vi "Divby3.vi"() -> ()   [LabVIEW 2020]
panel:
  out "Odd numbers divisible by 3":dbl[](array[numeric])
  out "Even numbers divisible by 3":dbl[](array[numeric])
  in  "Temp":dbl[](array[numeric])
  in  "Input  Array":dbl[](array[numeric])
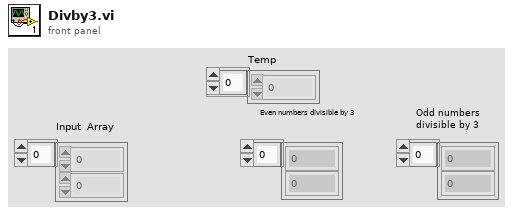
[diagram p1: front panel]
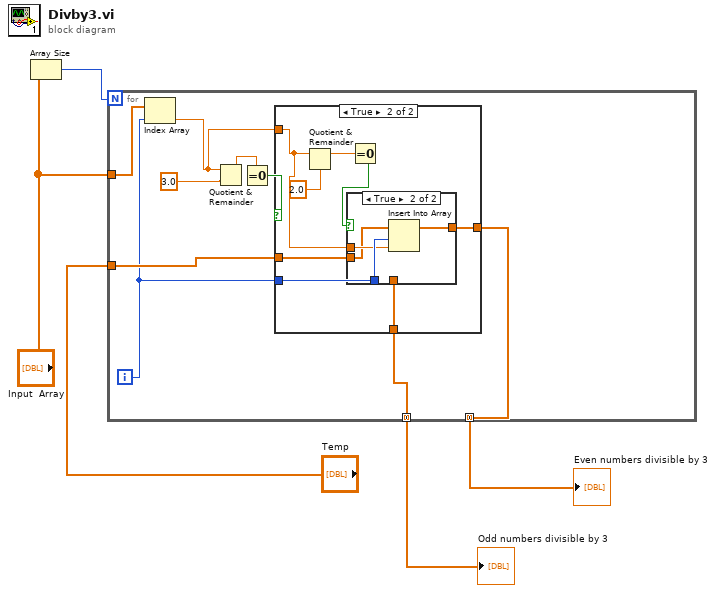
[diagram p0: block diagram]
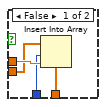
[diagram p3: hidden frame]
diagram:
  n1 = Array Size(array="Input  Array") -> (size(s)=w5:i32)
  n2 = for {
    N: w5 -> [_]
    tunnel: "Input  Array" -> [w14]
    tunnel: "Temp" -> [w9]
    tunnel: [w7] -> w2 mode=concatenating
    tunnel: [w6] -> w1 mode=concatenating
    i -> [w8]
    n3 = Index Array(array=w14, index=w8) -> (element=w10:dbl)
    n4 = Quotient & Remainder(x=w10, y=3.0) -> (x-y*floor(x/y)=w12:dbl)  [unwired: 1 out]
    n5 = Equal To 0?(x=w12) -> (x = 0?=w11:bool)
    n6 = case shown="True" w11 {
      tunnel: w10 -> [_ w17]
      tunnel: w9 -> [_ w19]
      tunnel: w8 -> [_ w18]
      tunnel: [_ w16] -> w7
      tunnel: [_ w15] -> w6
      frame False {
      }
      frame True {
        n7 = Quotient & Remainder(x=w17, y=2.0) -> (x-y*floor(x/y)=w21:dbl)  [unwired: 1 out]
        n8 = Equal To 0?(x=w21) -> (x = 0?=w20:bool)
        n9 = case shown="True" w20 {
          tunnel: w19 -> [w23 w27]
          tunnel: w18 -> [w24 w30]
          tunnel: w17 -> [w26 w29]
          tunnel: [w25 _] -> w16
          tunnel: [_ w28] -> w15
          frame False {
            n10 = Insert Into Array(array=w23, index=w24, new element=w26) -> (w25:dbl[])
          }
          frame True {
            n11 = Insert Into Array(array=w27, index=w30, new element=w29) -> (w28:dbl[])
          }
        }
      }
    }
  }
  "Even numbers divisible by 3" <- w1
  "Odd numbers divisible by 3" <- w2
